vi "Zmiana wartości.vi"(4 "Wartość":dbl) -> (1 "Zmiana wartości?":bool)   [LabVIEW 2012, in "Biblioteka moduł map v3.lvlib" / "Pomocnicze.lvlib"]
uses:
  Pomocnicze/Pomocnicze.lvlib
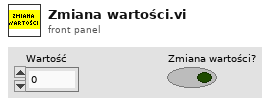
[diagram p1: front panel]
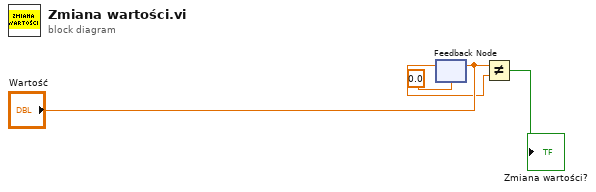
[diagram p0: block diagram]
diagram:
  n1 = feedback #1(0.0 ("Y")) -> (w1:dbl)
  n2 = feedback-in #1("Wartość") -> ()
  n3 = Not Equal?(x="Wartość", y=w1) -> (x != y?=→"Zmiana wartości?":bool)
